vi "Autonomous Independent.vi"() -> ()   [LabVIEW 2015]
doc: "This VI is called when autonomous begins, and will automatically be terminated when autonomous ends. You can carry out timed or sensor driven robot movement independently without needing to return to the caller."
uses:
  <vilib>/Rock Robotics/WPI/Utilities/WPI_GetSetVariantRefNum.vi
  <vilib>/Rock Robotics/Network Tables/NT Read String.vi
  Robot Global Data.vi
  <vilib>/Rock Robotics/WPI/RobotDrive/WPI_RobotDriveArcadeDrive_Standard(NoSaturation).vi
  <vilib>/Rock Robotics/Network Tables/NT Write Numeric Array.vi
panel:
  in  "Array of robot movements 5":T1(array[cluster])=[{"X Joystick Value"=0.0, "Y Joystick Value"=0.0, "Delay (sec)"=0.0, "Movement Name"="Stop", "Joystick Button 1"=FALSE, "Joystick Button 2"=FALSE, "Joystick Button 3"=FALSE, "Joystick Button 4"=FALSE, "Joystick Button 5"=FALSE, "Joystick Button 6"=FALSE, "Joystick Button 7"=FALSE, "Joystick Button 8"=FALSE, "Joystick Button 9"=FALSE, "Joystick Button 10"=FALSE, "Joystick Button 11"=FALSE, "Joystick Button 12"=FALSE}] {"Y Joystick Value" scale=1.0..-1.0; "X Joystick Value" scale=-1.0..1.0}
  in  "Array of robot movements 4":T1(array[cluster])=[{"X Joystick Value"=0.0, "Y Joystick Value"=0.5, "Delay (sec)"=1.0, "Movement Name"="Drive ", "Joystick Button 1"=FALSE, "Joystick Button 2"=FALSE, "Joystick Button 3"=FALSE, "Joystick Button 4"=FALSE, "Joystick Button 5"=FALSE, "Joystick Button 6"=FALSE, "Joystick Button 7"=FALSE, "Joystick Button 8"=FALSE, "Joystick Button 9"=FALSE, "Joystick Button 10"=FALSE, "Joystick Button 11"=FALSE, "Joystick Button 12"=FALSE}, {"X Joystick Value"=0.0, "Y Joystick Value"=0.0, "Delay (sec)"=3.0, "Movement Name"="Shoot", "Joystick Button 1"=TRUE, "Joystick Button 2"=FALSE, "Joystick Button 3"=FALSE, "Joystick Button 4"=FALSE, "Joystick Button 5"=FALSE, "Joystick Button 6"=FALSE, "Joystick Button 7"=FALSE, "Joystick Button 8"=FALSE, "Joystick Button 9"=FALSE, "Joystick Button 10"=FALSE, "Joystick Button 11"=FALSE, "Joystick Button 12"=FALSE}, {"X Joystick Value"=0.0, "Y Joystick Value"=0.0, "Delay (sec)"=0.0, "Movement Name"="Stop", "Joystick Button 1"=FALSE, "Joystick Button 2"=FALSE, "Joystick Button 3"=FALSE, "Joystick Button 4"=FALSE, "Joystick Button 5"=FALSE, "Joystick Button 6"=FALSE, "Joystick Button 7"=FALSE, "Joystick Button 8"=FALSE, "Joystick Button 9"=FALSE, "Joystick Button 10"=FALSE, "Joystick Button 11"=FALSE, "Joystick Button 12"=FALSE}] {"Y Joystick Value" scale=1.0..-1.0; "X Joystick Value" scale=-1.0..1.0}
  in  "Array of robot movements 3":T1(array[cluster])=[{"X Joystick Value"=0.0, "Y Joystick Value"=1.0, "Delay (sec)"=10.0, "Movement Name"="Drive", "Joystick Button 1"=FALSE, "Joystick Button 2"=FALSE, "Joystick Button 3"=FALSE, "Joystick Button 4"=FALSE, "Joystick Button 5"=FALSE, "Joystick Button 6"=FALSE, "Joystick Button 7"=FALSE, "Joystick Button 8"=FALSE, "Joystick Button 9"=FALSE, "Joystick Button 10"=FALSE, "Joystick Button 11"=FALSE, "Joystick Button 12"=FALSE}, {"X Joystick Value"=0.0, "Y Joystick Value"=0.0, "Delay (sec)"=0.0, "Movement Name"="Stop", "Joystick Button 1"=FALSE, "Joystick Button 2"=FALSE, "Joystick Button 3"=FALSE, "Joystick Button 4"=FALSE, "Joystick Button 5"=FALSE, "Joystick Button 6"=FALSE, "Joystick Button 7"=FALSE, "Joystick Button 8"=FALSE, "Joystick Button 9"=FALSE, "Joystick Button 10"=FALSE, "Joystick Button 11"=FALSE, "Joystick Button 12"=FALSE}] {"Y Joystick Value" scale=1.0..-1.0; "X Joystick Value" scale=-1.0..1.0}
  in  "Array of robot movements 2":T1(array[cluster])=[{"X Joystick Value"=0.0, "Y Joystick Value"=0.7, "Delay (sec)"=3.0, "Movement Name"="Low Mode + Drive", "Joystick Button 1"=FALSE, "Joystick Button 2"=FALSE, "Joystick Button 3"=FALSE, "Joystick Button 4"=FALSE, "Joystick Button 5"=FALSE, "Joystick Button 6"=FALSE, "Joystick Button 7"=TRUE, "Joystick Button 8"=FALSE, "Joystick Button 9"=FALSE, "Joystick Button 10"=FALSE, "Joystick Button 11"=FALSE, "Joystick Button 12"=FALSE}, {"X Joystick Value"=0.0, "Y Joystick Value"=0.0, "Delay (sec)"=3.0, "Movement Name"="Shoot", "Joystick Button 1"=TRUE, "Joystick Button 2"=FALSE, "Joystick Button 3"=FALSE, "Joystick Button 4"=FALSE, "Joystick Button 5"=FALSE, "Joystick Button 6"=FALSE, "Joystick Button 7"=FALSE, "Joystick Button 8"=FALSE, "Joystick Button 9"=FALSE, "Joystick Button 10"=FALSE, "Joystick Button 11"=FALSE, "Joystick Button 12"=FALSE}, {"X Joystick Value"=0.0, "Y Joystick Value"=0.0, "Delay (sec)"=0.0, "Movement Name"="Stop", "Joystick Button 1"=FALSE, "Joystick Button 2"=FALSE, "Joystick Button 3"=FALSE, "Joystick Button 4"=FALSE, "Joystick Button 5"=FALSE, "Joystick Button 6"=FALSE, "Joystick Button 7"=FALSE, "Joystick Button 8"=FALSE, "Joystick Button 9"=FALSE, "Joystick Button 10"=FALSE, "Joystick Button 11"=FALSE, "Joystick Button 12"=FALSE}] {"Y Joystick Value" scale=1.0..-1.0; "X Joystick Value" scale=-1.0..1.0}
  in  "Array of robot movements 1":T1(array[cluster])=[{"X Joystick Value"=0.0, "Y Joystick Value"=0.7, "Delay (sec)"=3.0, "Movement Name"="Low mode +Drive", "Joystick Button 1"=FALSE, "Joystick Button 2"=FALSE, "Joystick Button 3"=FALSE, "Joystick Button 4"=FALSE, "Joystick Button 5"=FALSE, "Joystick Button 6"=FALSE, "Joystick Button 7"=TRUE, "Joystick Button 8"=FALSE, "Joystick Button 9"=FALSE, "Joystick Button 10"=FALSE, "Joystick Button 11"=FALSE, "Joystick Button 12"=FALSE}, {"X Joystick Value"=0.5, "Y Joystick Value"=0.0, "Delay (sec)"=0.5, "Movement Name"="turn right 40 deg", "Joystick Button 1"=FALSE, "Joystick Button 2"=FALSE, "Joystick Button 3"=FALSE, "Joystick Button 4"=FALSE, "Joystick Button 5"=FALSE, "Joystick Button 6"=FALSE, "Joystick Button 7"=FALSE, "Joystick Button 8"=FALSE, "Joystick Button 9"=FALSE, "Joystick Button 10"=FALSE, "Joystick Button 11"=FALSE, "Joystick Button 12"=FALSE}, {"X Joystick Value"=0.0, "Y Joystick Value"=0.0, "Delay (sec)"=3.0, "Movement Name"="Shoot sequence", "Joystick Button 1"=TRUE, "Joystick Button 2"=FALSE, "Joystick Button 3"=FALSE, "Joystick Button 4"=FALSE, "Joystick Button 5"=FALSE, "Joystick Button 6"=FALSE, "Joystick Button 7"=FALSE, "Joystick Button 8"=FALSE, "Joystick Button 9"=FALSE, "Joystick Button 10"=FALSE, "Joystick Button 11"=FALSE, "Joystick Button 12"=FALSE}, {"X Joystick Value"=0.0, "Y Joystick Value"=0.0, "Delay (sec)"=0.0, "Movement Name"="Stop", "Joystick Button 1"=FALSE, "Joystick Button 2"=FALSE, "Joystick Button 3"=FALSE, "Joystick Button 4"=FALSE, "Joystick Button 5"=FALSE, "Joystick Button 6"=FALSE, "Joystick Button 7"=FALSE, "Joystick Button 8"=FALSE, "Joystick Button 9"=FALSE, "Joystick Button 10"=FALSE, "Joystick Button 11"=FALSE, "Joystick Button 12"=FALSE}] {"Y Joystick Value" scale=1.0..-1.0; "X Joystick Value" scale=-1.0..1.0}
  # "Be sure to right-click and choose Data Operations>>Make Current Value default if you want to save the array values with the VI"
  # "AUTO 1. LOW BAR"
  # "AUTO 2. DEFENCE 3"
  # "AUTO 3. TOUCH GOAL"
  # "AUTO 4. SPY BOT"
  # "AUTO 5. NOTHING"
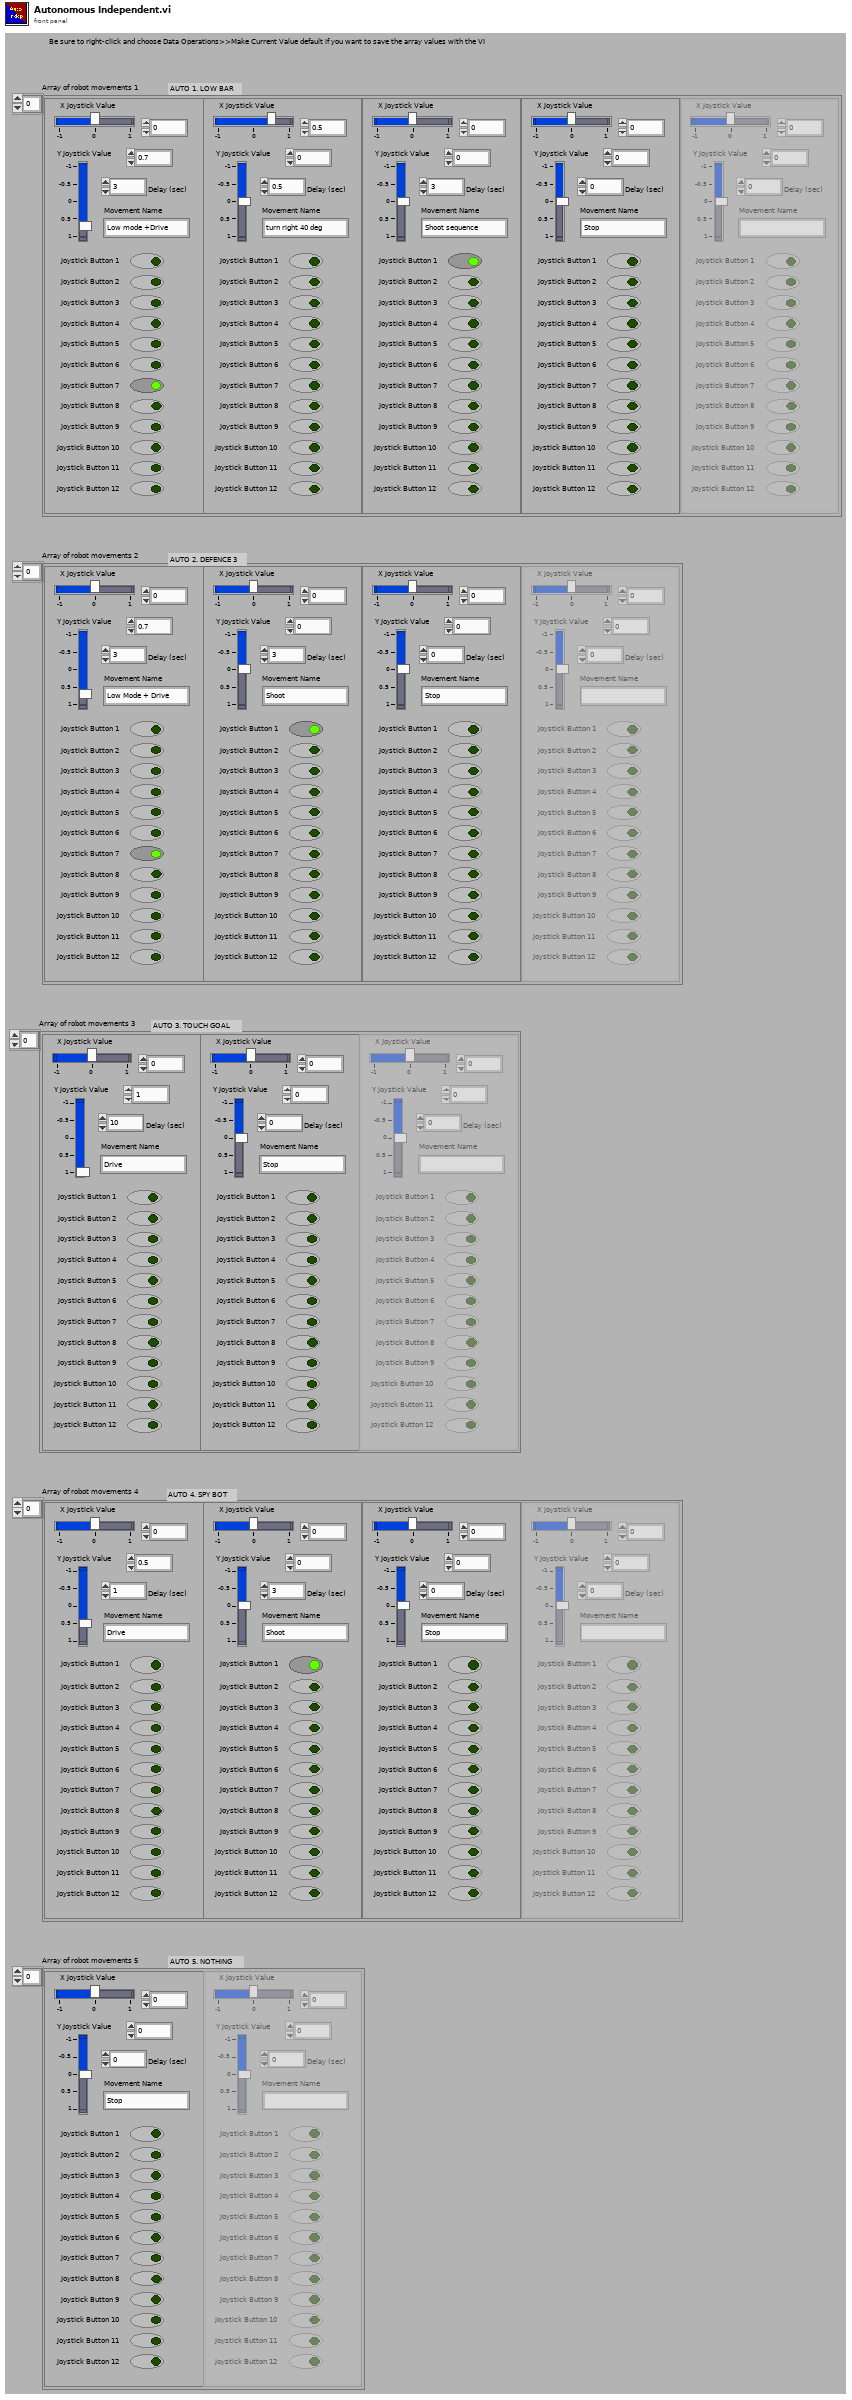
[diagram p1: front panel]
types:
  T1 = cluster{"X Joystick Value":dbl, "Y Joystick Value":dbl, "Delay (sec)":dbl, "Movement Name":string, "Joystick Button 1":bool, "Joystick Button 2":bool, "Joystick Button 3":bool, "Joystick Button 4":bool, "Joystick Button 5":bool, "Joystick Button 6":bool, "Joystick Button 7":bool, "Joystick Button 8":bool, "Joystick Button 9":bool, "Joystick Button 10":bool, "Joystick Button 11":bool, "Joystick Button 12":bool}[]
  T2 = typedef "WPI_JoystickDevRef.ctl" = cluster{"Device":T3}
  T3 = typedef "WPI_JoystickDeviceEnum.ctl" = enum16{"USB 0", "USB 1", "USB 2", "USB 3", "USB 4", "USB 5"}
  T4 = typedef "WPI_RobotDriveDevRef.ctl" = cluster{"DevStatus":errorcluster, "Motors[]":T5[], "Square Inputs":bool, "Max Output":dbl}
  T5 = typedef "WPI_MotorControlDeviceRef.ctl" = cluster{"DeviceStatus":errorcluster, "Type":T6, "PWM":cluster{"PWM Channel":T7, "DeadBand":T8}, "CAN":cluster{"Device Number":u8, "Control Mode":T9, "Semaphore":T10, "Max Vout":dbl, "TalonSRX Control Mode":T11}, "Invert":bool}
  T6 = typedef "WPI_MotorControlType.ctl" = enum16{"PWM", "CAN", "CANTalonSRX"}
  T7 = typedef "FPGA_DIOPWMChannel.ctl" = enum8{"PWM 0", "PWM 1", "PWM 2", "PWM 3", "PWM 4", "PWM 5", "PWM 6", "PWM 7", "PWM 8", "PWM 9", "PWM MXP 0", "PWM MXP 1", "PWM MXP 2", "PWM MXP 3", "PWM MXP 4", "PWM MXP 5", "PWM MXP 6", "PWM MXP 7", "PWM MXP 8", "PWM MXP 9", "Invalid"}
  T8 = typedef "WPI_PWMDeadband.ctl" = cluster{"Name":string, "maxPositivePwm":i32, "minPositivePwm":i32, "centerPwm":i32, "maxNegativePwm":i32, "minNegativePwm":i32, "angularRange":u16}
  T9 = typedef "WPI_CANJaguar_ControlMode.ctl" = enum8{"Percent VBus", "Current", "Speed", "Position", "Voltage"}
  T10 = typedef "Semaphore RefNum" = refnum<k1>
  T11 = typedef "WPI_CANTalonSRX_APIControlMode.ctl" = enum8{"Percent VBus", "Speed", "Position", "Slave", "Unchanged / Invalid", "Voltage Compensation", "Current", "Motion Profile"}
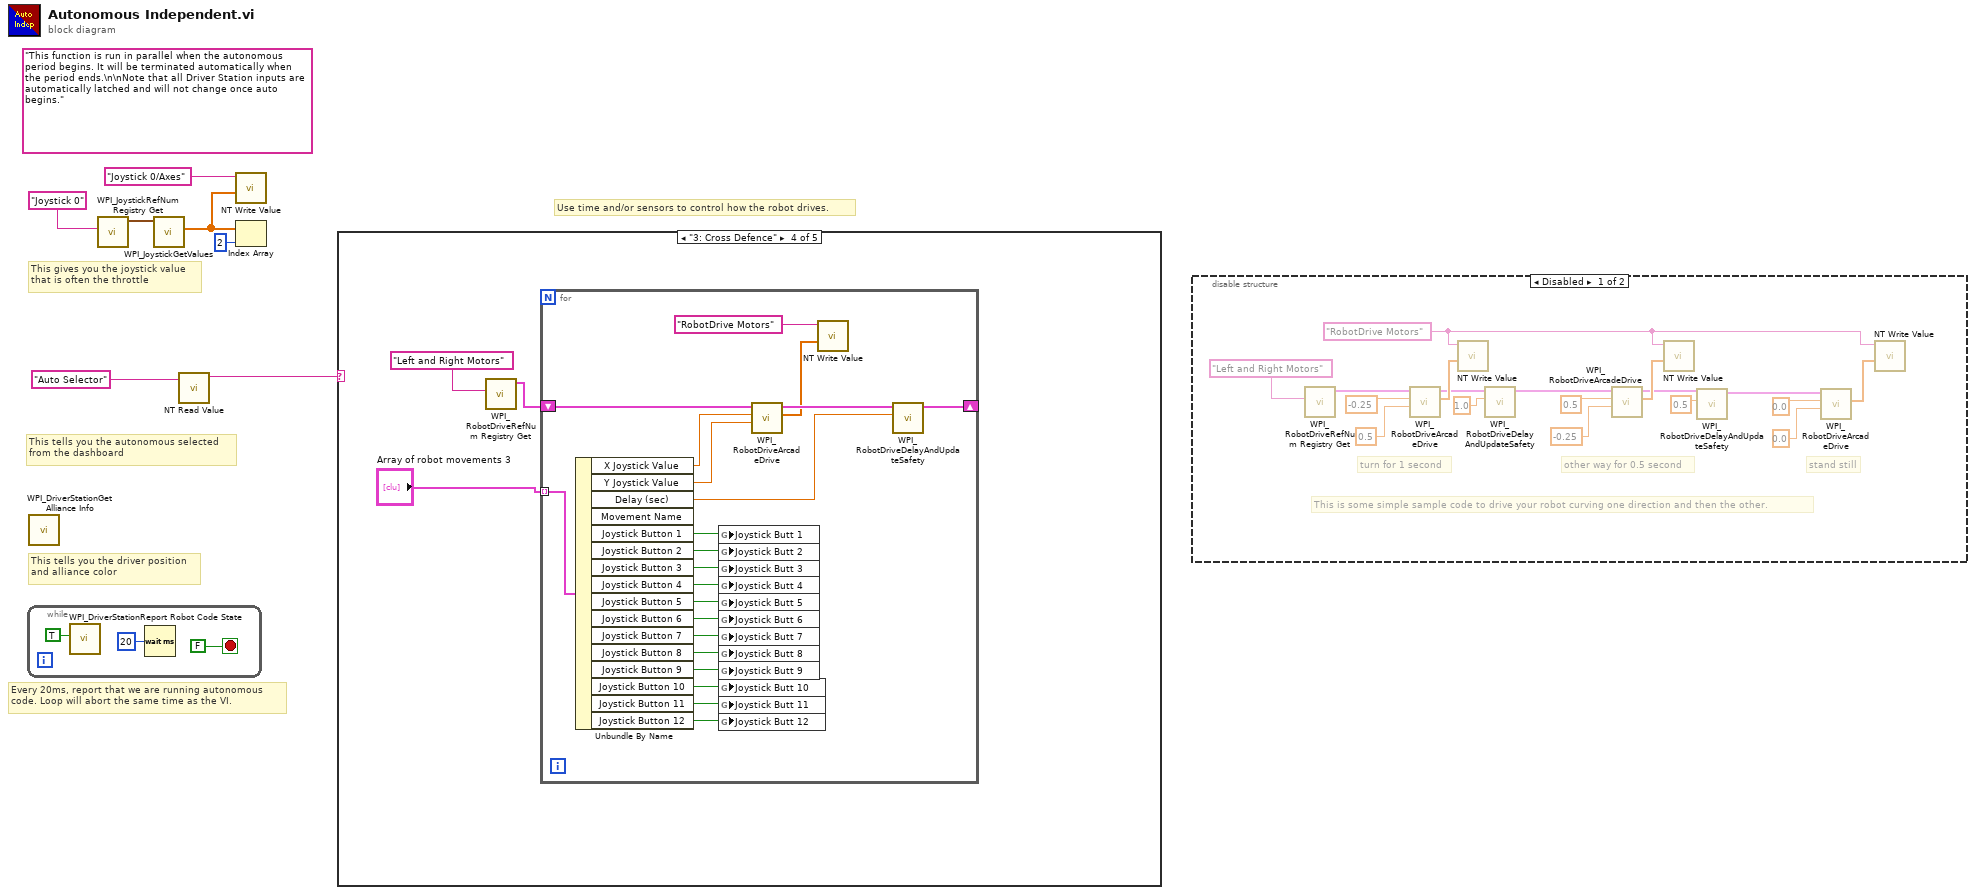
[diagram p0: block diagram]
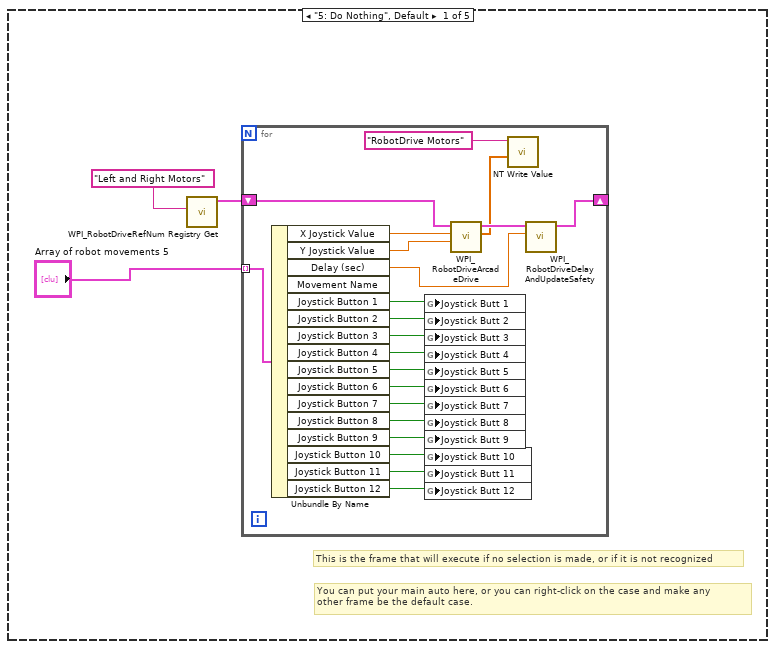
[diagram p3: hidden frame]
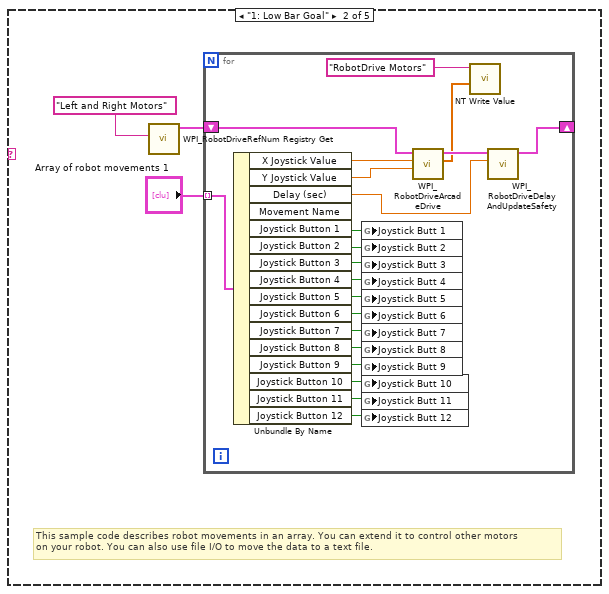
[diagram p4: hidden frame]
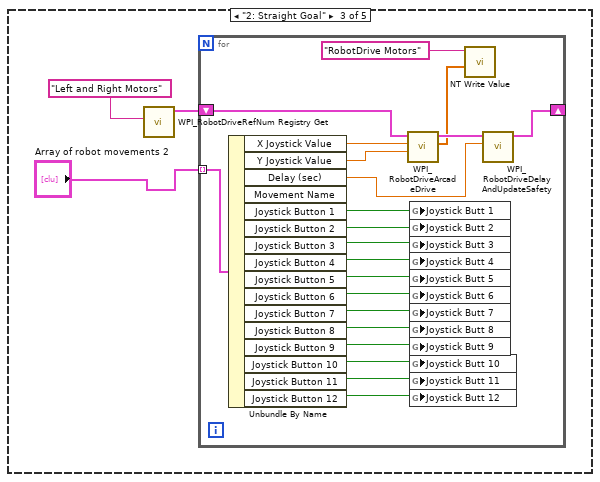
[diagram p5: hidden frame]
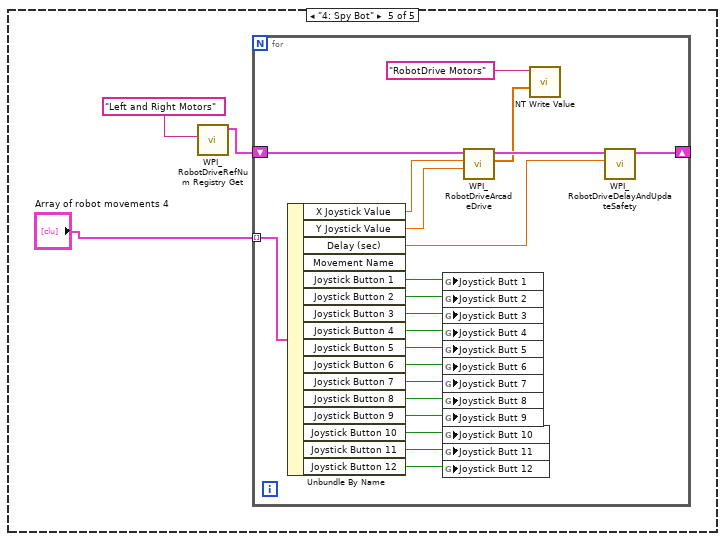
[diagram p6: hidden frame]
diagram:
  (unwired) "This function is run in parallel when the autonomous period begins. It will be terminated automatically when the period ends.\n\nNote that all Driver Station inputs are automatically latched and will not change once auto begins."
  # "This tells you the autonomous selected\nfrom the dashboard"
  # "Every 20ms, report that we are running autonomous\ncode. Loop will abort the same time as the VI."
  # "This gives you the joystick value\nthat is often the throttle"
  # "Use time and/or sensors to control how the robot drives."
  # "This tells you the driver position\nand alliance color"
  n1 = while {
    stop <- FALSE stop-if-true
    n2 = call <vilib>:"WPI_DriverStationReport Robot Code State.vi"("Autonomous"=TRUE) -> ()  [unwired: 10 in, 1 out]
    n3 = Wait (ms)(milliseconds to wait=u32 20) -> ()  [unwired: 1 out]
  }
  n4 = call <vilib>:"WPI_DriverStationGet Alliance Info.vi"() -> ()  [unwired: 12 out]
  n5 = call <vilib>:"WPI_JoystickRefNum Registry Get.vi"("refnum name"="Joystick 0") -> ("JoystickDevRef"=w6:T2)  [unwired: 1 in, 9 out]
  n6 = call <vilib>:"WPI_JoystickGetValues.vi"("JoystickDevRef"=w6) -> ("Axes"=w2:dbl[])  [unwired: 6 in, 4 out]
  n7 = call-poly <vilib>:"NT Read Value.vi"("Name"="Auto Selector") -> ("String"=w3:string)  [unwired: 9 in, 1 out]
  n8 = call-poly <vilib>:"NT Write Value.vi"("Numeric Array"=w2, "Name"="Joystick 0/Axes") -> ()  [unwired: 9 in, 1 out]
  n9 = Index Array(array=w2, index=2) -> ()  [unwired: 1 out]
  n10 = case shown="\"3: Cross Defence\"" w3 {
    frame "5: Do Nothing", Default {
      # "You can put your main auto here, or you can right-click on the case and make any\nother frame be the default case."
      # "This is the frame that will execute if no selection is made, or if it is not recognized"
      n11 = call <vilib>:"WPI_RobotDriveRefNum Registry Get.vi"("refnum name"="Left and Right Motors") -> ("RobotDriveDevRef"=w12:T4)  [unwired: 1 in, 9 out]
      n12 = for {
        shift-right: [w32] -> _
        shift-left: w12 -> [w33]
        tunnel: "Array of robot movements 5" -> [w28] mode=indexing
        n13 = Unbundle By Name(w28) -> ("X Joystick Value"=w31:dbl, "Y Joystick Value"=w30:dbl, "Delay (sec)"=w29:dbl, "Joystick Button 1"=w25:bool, "Joystick Button 2"=w24:bool, "Joystick Button 3"=w23:bool, "Joystick Button 4"=w22:bool, "Joystick Button 5"=w21:bool, "Joystick Button 6"=w20:bool, "Joystick Button 7"=w19:bool, "Joystick Button 8"=w18:bool, "Joystick Button 9"=w17:bool, "Joystick Button 10"=w16:bool, "Joystick Button 11"=w15:bool, "Joystick Button 12"=w14:bool)  [unwired: 1 out]
        n14 = global write "Robot Global Data.vi" "Joystick Butt 1"(w25) -> ()
        n15 = global write "Robot Global Data.vi" "Joystick Butt 2"(w24) -> ()
        n16 = global write "Robot Global Data.vi" "Joystick Butt 3"(w23) -> ()
        n17 = global write "Robot Global Data.vi" "Joystick Butt 4"(w22) -> ()
        n18 = global write "Robot Global Data.vi" "Joystick Butt 5"(w21) -> ()
        n19 = global write "Robot Global Data.vi" "Joystick Butt 6"(w20) -> ()
        n20 = global write "Robot Global Data.vi" "Joystick Butt 7"(w19) -> ()
        n21 = global write "Robot Global Data.vi" "Joystick Butt 8"(w18) -> ()
        n22 = global write "Robot Global Data.vi" "Joystick Butt 9"(w17) -> ()
        n23 = global write "Robot Global Data.vi" "Joystick Butt 10"(w16) -> ()
        n24 = global write "Robot Global Data.vi" "Joystick Butt 11"(w15) -> ()
        n25 = global write "Robot Global Data.vi" "Joystick Butt 12"(w14) -> ()
        n26 = call-poly <vilib>:"WPI_RobotDriveArcadeDrive.vi"("Y axis value"=w30, "X axis value"=w31, "RobotDriveDevRef"=w33) -> ("Motor Values"=w26:dbl[], "RobotDriveDevRef"=w34:T4)  [unwired: 1 in, 6 out]
        n27 = call-poly <vilib>:"NT Write Value.vi"("Numeric Array"=w26, "Name"="RobotDrive Motors") -> ()  [unwired: 9 in, 1 out]
        n28 = call <vilib>:"WPI_RobotDriveDelayAndUpdateSafety.vi"("Delay (s)"=w29, "RobotDriveDevRef"=w34) -> ("RobotDriveDevRef 2"=w32:T4)  [unwired: 8 in, 1 out]
      }
    }
    frame "1: Low Bar Goal" {
      # "This sample code describes robot movements in an array. You can extend it to control other motors\non your robot. You can also use file I/O to move the data to a text file."
      n29 = call <vilib>:"WPI_RobotDriveRefNum Registry Get.vi"("refnum name"="Left and Right Motors") -> ("RobotDriveDevRef"=w36:T4)  [unwired: 1 in, 9 out]
      n30 = for {
        shift-right: [w56] -> _
        shift-left: w36 -> [w57]
        tunnel: "Array of robot movements 1" -> [w52] mode=indexing
        n31 = Unbundle By Name(w52) -> ("X Joystick Value"=w55:dbl, "Y Joystick Value"=w54:dbl, "Delay (sec)"=w53:dbl, "Joystick Button 1"=w49:bool, "Joystick Button 2"=w48:bool, "Joystick Button 3"=w47:bool, "Joystick Button 4"=w46:bool, "Joystick Button 5"=w45:bool, "Joystick Button 6"=w44:bool, "Joystick Button 7"=w43:bool, "Joystick Button 8"=w42:bool, "Joystick Button 9"=w41:bool, "Joystick Button 10"=w40:bool, "Joystick Button 11"=w39:bool, "Joystick Button 12"=w38:bool)  [unwired: 1 out]
        n32 = global write "Robot Global Data.vi" "Joystick Butt 1"(w49) -> ()
        n33 = global write "Robot Global Data.vi" "Joystick Butt 2"(w48) -> ()
        n34 = global write "Robot Global Data.vi" "Joystick Butt 3"(w47) -> ()
        n35 = global write "Robot Global Data.vi" "Joystick Butt 4"(w46) -> ()
        n36 = global write "Robot Global Data.vi" "Joystick Butt 5"(w45) -> ()
        n37 = global write "Robot Global Data.vi" "Joystick Butt 6"(w44) -> ()
        n38 = global write "Robot Global Data.vi" "Joystick Butt 7"(w43) -> ()
        n39 = global write "Robot Global Data.vi" "Joystick Butt 8"(w42) -> ()
        n40 = global write "Robot Global Data.vi" "Joystick Butt 9"(w41) -> ()
        n41 = global write "Robot Global Data.vi" "Joystick Butt 10"(w40) -> ()
        n42 = global write "Robot Global Data.vi" "Joystick Butt 11"(w39) -> ()
        n43 = global write "Robot Global Data.vi" "Joystick Butt 12"(w38) -> ()
        n44 = call-poly <vilib>:"WPI_RobotDriveArcadeDrive.vi"("Y axis value"=w54, "X axis value"=w55, "RobotDriveDevRef"=w57) -> ("Motor Values"=w50:dbl[], "RobotDriveDevRef"=w58:T4)  [unwired: 1 in, 6 out]
        n45 = call-poly <vilib>:"NT Write Value.vi"("Numeric Array"=w50, "Name"="RobotDrive Motors") -> ()  [unwired: 9 in, 1 out]
        n46 = call <vilib>:"WPI_RobotDriveDelayAndUpdateSafety.vi"("Delay (s)"=w53, "RobotDriveDevRef"=w58) -> ("RobotDriveDevRef 2"=w56:T4)  [unwired: 8 in, 1 out]
      }
    }
    frame "2: Straight Goal" {
      n47 = call <vilib>:"WPI_RobotDriveRefNum Registry Get.vi"("refnum name"="Left and Right Motors") -> ("RobotDriveDevRef"=w60:T4)  [unwired: 1 in, 9 out]
      n48 = for {
        shift-right: [w80] -> _
        shift-left: w60 -> [w81]
        tunnel: "Array of robot movements 2" -> [w76] mode=indexing
        n49 = Unbundle By Name(w76) -> ("X Joystick Value"=w79:dbl, "Y Joystick Value"=w78:dbl, "Delay (sec)"=w77:dbl, "Joystick Button 1"=w62:bool, "Joystick Button 2"=w63:bool, "Joystick Button 3"=w64:bool, "Joystick Button 4"=w65:bool, "Joystick Button 5"=w66:bool, "Joystick Button 6"=w67:bool, "Joystick Button 7"=w68:bool, "Joystick Button 8"=w69:bool, "Joystick Button 9"=w70:bool, "Joystick Button 10"=w71:bool, "Joystick Button 11"=w72:bool, "Joystick Button 12"=w73:bool)  [unwired: 1 out]
        n50 = call-poly <vilib>:"WPI_RobotDriveArcadeDrive.vi"("Y axis value"=w78, "X axis value"=w79, "RobotDriveDevRef"=w81) -> ("Motor Values"=w74:dbl[], "RobotDriveDevRef"=w82:T4)  [unwired: 1 in, 6 out]
        n51 = global write "Robot Global Data.vi" "Joystick Butt 1"(w62) -> ()
        n52 = global write "Robot Global Data.vi" "Joystick Butt 2"(w63) -> ()
        n53 = global write "Robot Global Data.vi" "Joystick Butt 3"(w64) -> ()
        n54 = global write "Robot Global Data.vi" "Joystick Butt 4"(w65) -> ()
        n55 = global write "Robot Global Data.vi" "Joystick Butt 5"(w66) -> ()
        n56 = global write "Robot Global Data.vi" "Joystick Butt 6"(w67) -> ()
        n57 = global write "Robot Global Data.vi" "Joystick Butt 7"(w68) -> ()
        n58 = global write "Robot Global Data.vi" "Joystick Butt 8"(w69) -> ()
        n59 = global write "Robot Global Data.vi" "Joystick Butt 9"(w70) -> ()
        n60 = global write "Robot Global Data.vi" "Joystick Butt 10"(w71) -> ()
        n61 = global write "Robot Global Data.vi" "Joystick Butt 11"(w72) -> ()
        n62 = global write "Robot Global Data.vi" "Joystick Butt 12"(w73) -> ()
        n63 = call-poly <vilib>:"NT Write Value.vi"("Numeric Array"=w74, "Name"="RobotDrive Motors") -> ()  [unwired: 9 in, 1 out]
        n64 = call <vilib>:"WPI_RobotDriveDelayAndUpdateSafety.vi"("Delay (s)"=w77, "RobotDriveDevRef"=w82) -> ("RobotDriveDevRef 2"=w80:T4)  [unwired: 8 in, 1 out]
      }
    }
    frame "3: Cross Defence" {
      n65 = call <vilib>:"WPI_RobotDriveRefNum Registry Get.vi"("refnum name"="Left and Right Motors") -> ("RobotDriveDevRef"=w84:T4)  [unwired: 1 in, 9 out]
      n66 = for {
        tunnel: "Array of robot movements 3" -> [w106] mode=indexing
        shift-right: [w98] -> _
        shift-left: w84 -> [w105]
        n67 = Unbundle By Name(w106) -> ("X Joystick Value"=w104:dbl, "Y Joystick Value"=w103:dbl, "Delay (sec)"=w99:dbl, "Joystick Button 1"=w97:bool, "Joystick Button 2"=w96:bool, "Joystick Button 3"=w95:bool, "Joystick Button 4"=w94:bool, "Joystick Button 5"=w93:bool, "Joystick Button 6"=w92:bool, "Joystick Button 7"=w91:bool, "Joystick Button 8"=w90:bool, "Joystick Button 9"=w89:bool, "Joystick Button 10"=w88:bool, "Joystick Button 11"=w87:bool, "Joystick Button 12"=w86:bool)  [unwired: 1 out]
        n68 = global write "Robot Global Data.vi" "Joystick Butt 1"(w97) -> ()
        n69 = global write "Robot Global Data.vi" "Joystick Butt 2"(w96) -> ()
        n70 = global write "Robot Global Data.vi" "Joystick Butt 3"(w95) -> ()
        n71 = global write "Robot Global Data.vi" "Joystick Butt 4"(w94) -> ()
        n72 = global write "Robot Global Data.vi" "Joystick Butt 5"(w93) -> ()
        n73 = global write "Robot Global Data.vi" "Joystick Butt 6"(w92) -> ()
        n74 = global write "Robot Global Data.vi" "Joystick Butt 7"(w91) -> ()
        n75 = global write "Robot Global Data.vi" "Joystick Butt 8"(w90) -> ()
        n76 = global write "Robot Global Data.vi" "Joystick Butt 9"(w89) -> ()
        n77 = global write "Robot Global Data.vi" "Joystick Butt 10"(w88) -> ()
        n78 = global write "Robot Global Data.vi" "Joystick Butt 11"(w87) -> ()
        n79 = global write "Robot Global Data.vi" "Joystick Butt 12"(w86) -> ()
        n80 = call-poly <vilib>:"WPI_RobotDriveArcadeDrive.vi"("Y axis value"=w103, "X axis value"=w104, "RobotDriveDevRef"=w105) -> ("Motor Values"=w100:dbl[], "RobotDriveDevRef"=w102:T4)  [unwired: 1 in, 6 out]
        n81 = call-poly <vilib>:"NT Write Value.vi"("Numeric Array"=w100, "Name"="RobotDrive Motors") -> ()  [unwired: 9 in, 1 out]
        n82 = call <vilib>:"WPI_RobotDriveDelayAndUpdateSafety.vi"("Delay (s)"=w99, "RobotDriveDevRef"=w102) -> ("RobotDriveDevRef 2"=w98:T4)  [unwired: 8 in, 1 out]
      }
    }
    frame "4: Spy Bot" {
      n83 = call <vilib>:"WPI_RobotDriveRefNum Registry Get.vi"("refnum name"="Left and Right Motors") -> ("RobotDriveDevRef"=w108:T4)  [unwired: 1 in, 9 out]
      n84 = for {
        tunnel: "Array of robot movements 4" -> [w130] mode=indexing
        shift-right: [w122] -> _
        shift-left: w108 -> [w129]
        n85 = Unbundle By Name(w130) -> ("X Joystick Value"=w128:dbl, "Y Joystick Value"=w127:dbl, "Delay (sec)"=w123:dbl, "Joystick Button 1"=w121:bool, "Joystick Button 2"=w120:bool, "Joystick Button 3"=w119:bool, "Joystick Button 4"=w118:bool, "Joystick Button 5"=w117:bool, "Joystick Button 6"=w116:bool, "Joystick Button 7"=w115:bool, "Joystick Button 8"=w114:bool, "Joystick Button 9"=w113:bool, "Joystick Button 10"=w112:bool, "Joystick Button 11"=w111:bool, "Joystick Button 12"=w110:bool)  [unwired: 1 out]
        n86 = global write "Robot Global Data.vi" "Joystick Butt 1"(w121) -> ()
        n87 = global write "Robot Global Data.vi" "Joystick Butt 2"(w120) -> ()
        n88 = global write "Robot Global Data.vi" "Joystick Butt 3"(w119) -> ()
        n89 = global write "Robot Global Data.vi" "Joystick Butt 4"(w118) -> ()
        n90 = global write "Robot Global Data.vi" "Joystick Butt 5"(w117) -> ()
        n91 = global write "Robot Global Data.vi" "Joystick Butt 6"(w116) -> ()
        n92 = global write "Robot Global Data.vi" "Joystick Butt 7"(w115) -> ()
        n93 = global write "Robot Global Data.vi" "Joystick Butt 8"(w114) -> ()
        n94 = global write "Robot Global Data.vi" "Joystick Butt 9"(w113) -> ()
        n95 = global write "Robot Global Data.vi" "Joystick Butt 10"(w112) -> ()
        n96 = global write "Robot Global Data.vi" "Joystick Butt 11"(w111) -> ()
        n97 = global write "Robot Global Data.vi" "Joystick Butt 12"(w110) -> ()
        n98 = call-poly <vilib>:"WPI_RobotDriveArcadeDrive.vi"("Y axis value"=w127, "X axis value"=w128, "RobotDriveDevRef"=w129) -> ("Motor Values"=w124:dbl[], "RobotDriveDevRef"=w126:T4)  [unwired: 1 in, 6 out]
        n99 = call-poly <vilib>:"NT Write Value.vi"("Numeric Array"=w124, "Name"="RobotDrive Motors") -> ()  [unwired: 9 in, 1 out]
        n100 = call <vilib>:"WPI_RobotDriveDelayAndUpdateSafety.vi"("Delay (s)"=w123, "RobotDriveDevRef"=w126) -> ("RobotDriveDevRef 2"=w122:T4)  [unwired: 8 in, 1 out]
      }
    }
  }
  n101 = disable-structure shown="Disabled" {
    frame Disabled {
      w147 = "RobotDrive Motors" ("Name")
      # "This is some simple sample code to drive your robot curving one direction and then the other."
      # "stand still"
      # "other way for 0.5 second"
      # "turn for 1 second"
      n102 = call <vilib>:"WPI_RobotDriveRefNum Registry Get.vi"("refnum name"="Left and Right Motors") -> ("RobotDriveDevRef"=w131:T4)  [unwired: 1 in, 9 out]
      n103 = call-poly <vilib>:"WPI_RobotDriveArcadeDrive.vi"("Y axis value"=0.5 ("X axis value"), "X axis value"=-0.25, "RobotDriveDevRef"=w131) -> ("Motor Values"=w148:dbl[], "RobotDriveDevRef"=w138:T4)  [unwired: 1 in, 6 out]
      n104 = call-poly <vilib>:"NT Write Value.vi"("Numeric Array"=w148, "Name"=w147) -> ()  [unwired: 9 in, 1 out]
      n105 = call <vilib>:"WPI_RobotDriveDelayAndUpdateSafety.vi"("Delay (s)"=1.0, "RobotDriveDevRef"=w138) -> ("RobotDriveDevRef 2"=w137:T4)  [unwired: 8 in, 1 out]
      n106 = call-poly <vilib>:"WPI_RobotDriveArcadeDrive.vi"("Y axis value"=-0.25 ("X axis value"), "X axis value"=0.5, "RobotDriveDevRef"=w137) -> ("Motor Values"=w146:dbl[], "RobotDriveDevRef"=w136:T4)  [unwired: 1 in, 6 out]
      n107 = call-poly <vilib>:"NT Write Value.vi"("Numeric Array"=w146, "Name"=w147) -> ()  [unwired: 9 in, 1 out]
      n108 = call <vilib>:"WPI_RobotDriveDelayAndUpdateSafety.vi"("Delay (s)"=0.5, "RobotDriveDevRef"=w136) -> ("RobotDriveDevRef 2"=w135:T4)  [unwired: 8 in, 1 out]
      n109 = call-poly <vilib>:"WPI_RobotDriveArcadeDrive.vi"("Y axis value"=0.0 ("X axis value"), "X axis value"=0.0, "RobotDriveDevRef"=w135) -> ("Motor Values"=w145:dbl[])  [unwired: 1 in, 7 out]
      n110 = call-poly <vilib>:"NT Write Value.vi"("Numeric Array"=w145, "Name"=w147) -> ()  [unwired: 9 in, 1 out]
    }
    frame Enabled {
    }
  }
